vi "Test Case, Process File.vi"(8 "error in":errorcluster) -> (0 "error out":errorcluster, 1 "Input Parameters":T1[](array[typedef]) {"Value" format="%#.3f"}, 2 "Results":T1[](array[typedef]) {"Value" format="%#.3f"}, 3 "waveform filtered":waveform(dbl)(graph)={"t0"=timestamp(3472747248.0780005 s since 1904-01-01), "dt"=2e-06, "Y"=[]})   [LabVIEW 2010]
uses:
  Generic/Waveform Attribute/Waveform Attribute Cluster.ctl
panel:
  in  "Use Average Size from Waveform":bool=TRUE
  in  "Use Resistance from Waveform":bool=TRUE
  out "Average Size\n[from waveform]":dbl
  out "Resistance (ohms)\n[from waveform]":dbl
  in  "Average Size":dbl=15.0
  in  "Resistance (ohms)":dbl=500.0 format="%.1f"
  in  "Waveform Filtered Zoom":bool=TRUE
  in  "Waveform Zoom":bool
  in  "filename":path=path "C:/5-01-003 Active Electrode Min Max/Waveform 3 -10 mA"
  out "waveform":waveform(dbl)(graph)={"t0"=timestamp(3473168095.069 s since 1904-01-01), "dt"=2e-06, "Y"=[]}
  out "waveform array":waveform(dbl)={"t0"=timestamp(-9593225999.921999 s since 1904-01-01), "dt"=nan, "Y"=[]}
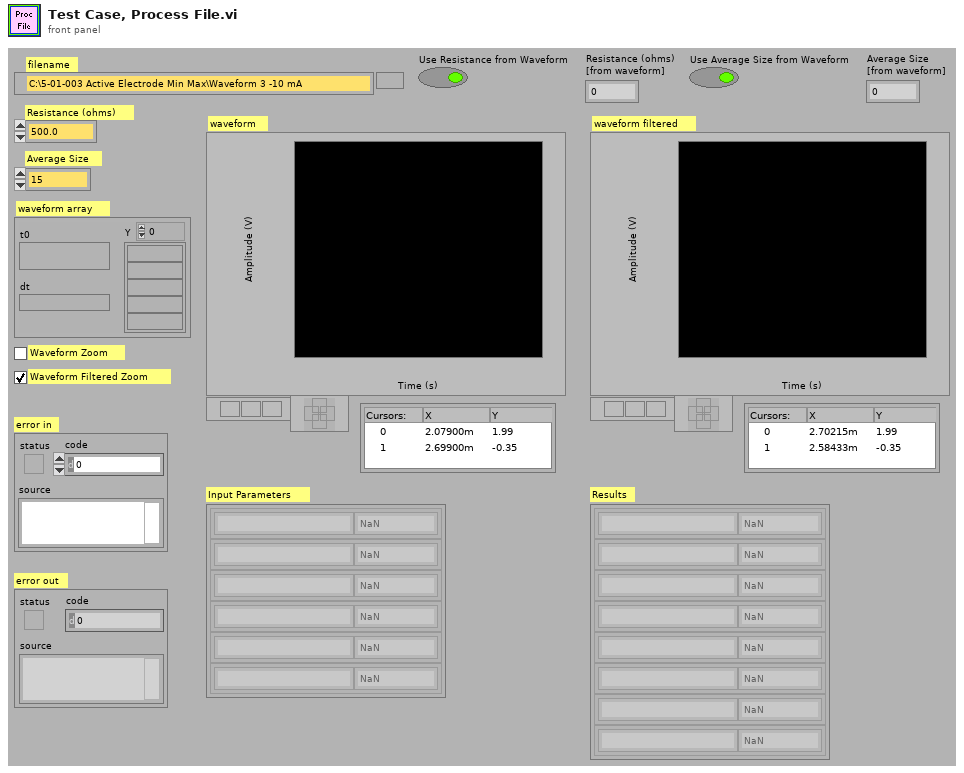
[diagram p1: front panel]
types:
  T1 = typedef "Waveform Attribute Cluster.ctl" = cluster{"Label":string, "Value":dbl}
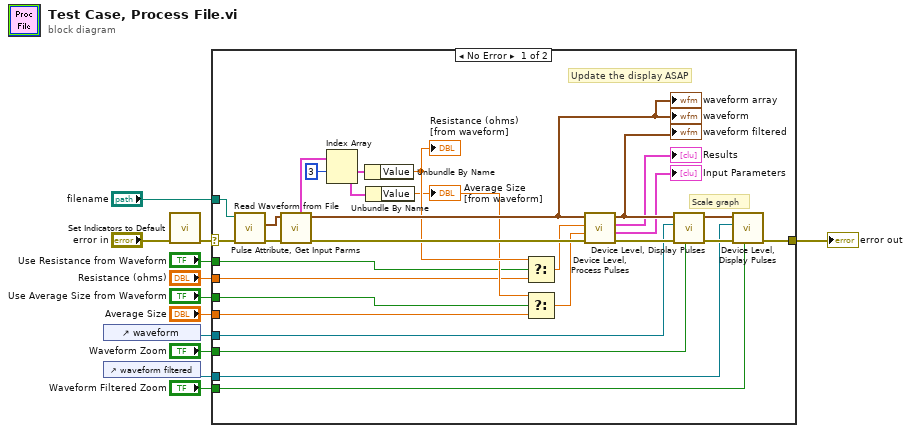
[diagram p0: block diagram]
diagram:
  n1 = control-ref of="waveform"() -> (w11:refnum<vi>)
  n2 = control-ref of="waveform filtered"() -> (w10:refnum<vi>)
  n3 = call "Set Indicators to Default.vi"("error in"="error in") -> ("error out"=w1:errorcluster)  [unwired: 6 in]
  n4 = case shown="No Error" w1 {
    selector: w1 -> [w33 w42]
    tunnel: [w32 w42] -> w12
    tunnel: w11 -> [w38 _]
    tunnel: w10 -> [w37 _]
    tunnel: "Waveform Zoom" -> [w36 _]
    tunnel: "Waveform Filtered Zoom" -> [w35 _]
    tunnel: "Resistance (ohms)" -> [w16 _]
    tunnel: "Average Size" -> [w15 _]
    tunnel: "filename" -> [w31 _]
    tunnel: "Use Resistance from Waveform" -> [w14 _]
    tunnel: "Use Average Size from Waveform" -> [w13 _]
    frame No Error {
      # "Update the display ASAP"
      # "Scale graph"
      n5 = call <vilib>:"Read Waveform from File.vi"("error in (no error)"=w33, "file path (dialog if empty)"=w31) -> ("error out"=w27:errorcluster, "first waveform in record"=w28:waveform(dbl))  [unwired: 4 in, 2 out]
      n6 = call "Pulse Attribute, Get Input Parms.vi"("error in"=w27, "waveform"=w28) -> ("error out"=w26:errorcluster, "waveform dup"=w25:waveform(dbl), "input parameters"=w24:T1[])  [unwired: 5 in]
      "waveform array" <- w25
      "waveform" <- w25
      n7 = Index Array(array=w24, index #1=3 ("index")) -> (element #1=w22:T1, element #2=w21:T1)  [unwired: 1 in]
      n8 = Unbundle By Name(w22) -> ("Value"=w20:dbl)
      "Resistance (ohms)\n[from waveform]" <- w20
      n9 = Unbundle By Name(w21) -> ("Value"=w18:dbl)
      "Average Size\n[from waveform]" <- w18
      n10 = Select(t=w20, s=w14, f=w16) -> (s? t:f=w19:dbl)
      n11 = Select(t=w18, s=w13, f=w15) -> (s? t:f=w17:dbl)
      n12 = call "Device Level, Process Pulses.vi"("error in"=w26, "Average Size"=w17, "Resistance (ohms)"=w19, "waveform"=w25) -> ("error out"=w41:errorcluster, "Input Parameters"=→"Input Parameters":T1[], "Results"=→"Results":T1[], "waveform out"=w34:waveform(dbl))  [unwired: 2 in]
      "waveform filtered" <- w34
      n13 = call "Device Level, Display Pulses.vi"("error in"=w41, "WFGraph Refnum"=w38, "waveform"=w34, "Zoom (F)"=w36) -> ("error out"=w40:errorcluster, "waveform dup"=w39:waveform(dbl))  [unwired: 5 in]
      n14 = call "Device Level, Display Pulses.vi"("error in"=w40, "WFGraph Refnum"=w37, "waveform"=w39, "Zoom (F)"=w35) -> ("error out"=w32:errorcluster)  [unwired: 5 in, 1 out]
    }
    frame Error {
    }
  }
  "error out" <- w12
